vi "Traverse_Sub_Read_Position.vi"(8 "error in (no error)":errorcluster, 11 "Network Path":string="192.168.1.52,1,0") -> (0 "error out":errorcluster, 1 "z position mm":sgl format="%_10g", 2 "y position mm":sgl format="%_10g", 3 "x position mm":sgl format="%_10g")   [LabVIEW 2018]
uses:
  <vilib>/ethernetip/ethernetip.llb/EthernetIP Tag Read REAL.vi
  <vilib>/ethernetip/ethernetip.lvlib
panel:
  in  "Tab Control":enum32{"Code Info", "Read Data", "Debug"}(tab)
  # "This code reads the current position of all three anemometer traverse axes in mm using Ethernet IP.\n\nIt will execute 1 time every time it is called.\n\nDO NOT CHANGE THE NETWORK ADDRESS!\n\nValues are polled directly from the PLC.\n\nDeveloped by Curtis Libby, 07/06/2021"
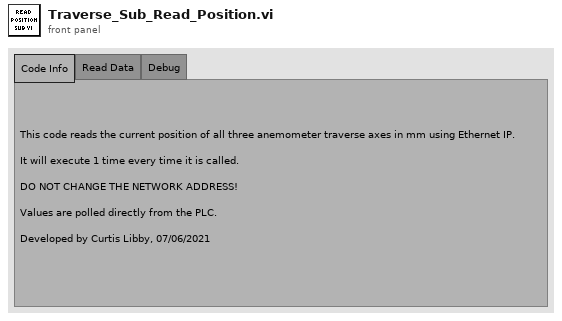
[diagram p1: front panel]
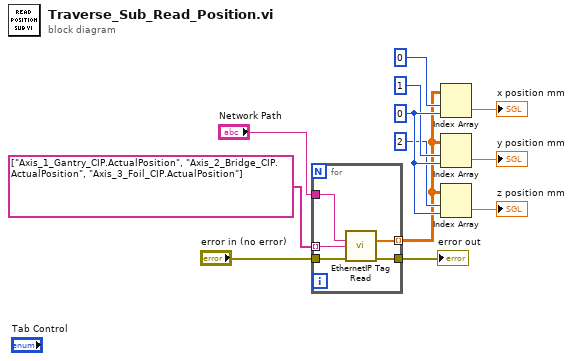
[diagram p0: block diagram]
diagram:
  w7 = 0 ("disabled index (col)")
  n1 = for {
    tunnel: string[] ["Axis_1_Gantry_CIP.ActualPosition", "Axis_2_Bridge_CIP.ActualPosition", "Axis_3_Foil_CIP.ActualPosition"] -> [w17] mode=indexing
    tunnel: [w16] -> w4 mode=indexing
    tunnel: "Network Path" -> [w15]
    tunnel: "error in (no error)" -> [w14]
    tunnel: [w13] -> w2
    n2 = call-poly <vilib>:"EthernetIP Tag Read.vi"("Network Path"=w15, "Tag Name"=w17, "error in"=w14) -> ("Data"=w16:sgl[], "error out"=w13:errorcluster)  [unwired: 10 in, 1 out]
  }
  "error out" <- w2
  n3 = Index Array(array=w4, index (row)=0, index (col)=w7) -> (element=→"x position mm":sgl)
  n4 = Index Array(array=w4, index (row)=1, index (col)=w7) -> (element=→"y position mm":sgl)
  n5 = Index Array(array=w4, index (row)=2, index (col)=w7) -> (element=→"z position mm":sgl)
